vi "AlliGator Generic Graph Actions.vi"(0 "AlliGator Q Elements in":T6[](array[typedef]), 1 "VI in":refnum<vi>, 2 "Script":bool, 5 "data value reference in":refnum<data-value>, 7 "AlliGator Q Event in":T7=enum."GUI:Idle", 9 "Data":variant, 11 "error in (no error)":errorcluster, 12 "AlliGator Ctrl Refnums":T8) -> (3 "Script out":bool, 4 "AlliGator Q Elements out":T6[](array[typedef]), 6 "Data Value Reference out":refnum<data-value>, 10 "[Notebook Message]":T1[](array[typedef]) {"Message Style"."Font Size" min=6.0 step=1.0}, 15 "error out":errorcluster)   [LabVIEW 2021, in "AlliGator Action Engine.lvlib"]
doc: "Processes AlliGator generic graph-related actions."
uses:
  AlliGator Action Engine.lvlib
  Internal Variables/AlliGator Internal Variables v2.ctl
  <vilib>/vision/Image Controls.llb/IMAQ Image.ctl
  Internal Variables/AlliGator Gate Image Set.ctl
  Files/AlliGator FLI Dataset Type.ctl
  Files/AlliGator Data Series Type.ctl
  Dual-Channel Datasets/AlliGator Dataset Channel.ctl
  Settings/AlliGator Gate Arithmetic.ctl
  Source Image/AlliGator Displayed Image.ctl
  Image/Named ROI Description.ctl
  Phasor Graph/AlliGator Decay Metadata v3.ctl
  Decay Analysis/Decay Preprocessing/AlliGator Decay Background Subtraction Info.ctl
  Decay Analysis/Decay Preprocessing/AlliGator Baseline Subtraction Method.ctl
  Graphs/XY Graph/XY Graph Plot Shift Parameters.ctl
  Graphs/XY Graph/XY Graph Plot Shift Method.ctl
  Decay Analysis/Decay Preprocessing/AlliGator Decay Extrapolation Parameters.ctl
  Phasor/Calibration Phasor (m, phi).ctl
  Phasor/Phasor Reference Series.ctl
  Phasor/Phasor Calibration Map v2.ctl
  Phasor/Phasor (g, s).ctl
  Phasor Graph/AlliGator Raw Phasor Plot Data v5.ctl
  Phasor/Phasor Standard Deviation Options.ctl
  Phasor Plot/AlliGator Phasor Multi-Harmonic Data.ctl
  Phasor/Phasor Harmonic Data.ctl
  Decay Fit Parameter Map/AlliGator Decay Fit Options & Parameters v3.ctl
  Fits/IRF(X)PSED/Decay Fit Options v3.ctl
  Fits/Decay Convolution/Decay Model.ctl
  Fits/Residual Type.ctl
  Fits/IRF(X)PSED/Fit Weights Type.ctl
  Fits/Non-linear Fitting Method v2.ctl
  Fits/Fit Calculation Method.ctl
  Fits/Non-linear Fitting Algorithm.ctl
  Decay Analysis/Decay Fit/AlliGator Decay Fit Parameter Constraints 2.ctl
  Fits/IRF(X)PSED/Decay Fit Parameters In List.ctl
  Fits/IRF(X)PSED/MLE Baseline Offset Type.ctl
  Decay Analysis/Decay Preprocessing/AlliGator Decay Preprocessing Parameters.ctl
  Fits/IRF(X)PSED/Decay Fit Parameters & Derived Quantities List v2.ctl
  Fits/IRF(X)PSED/Decay Fit Result Constraint.ctl
  Decay Fit Parameter Map/AlliGator Parameter Maps Data.ctl
  AlliGator Q Event.ctl
  GUI/AlliGator Ctrl Refnums.ctl
  GUI/AlliGator Other Ctrl Refnums.ctl
  GUI/AlliGator State Indicator.ctl
  GUI/AlliGator Main Window Tabs.ctl
  GUI/AlliGator Phasor Plot Ctrl Refnums.ctl
  GUI/AlliGator Phasor Graph Ctrl Refnums.ctl
  Phasor/Phasor Calibration Type.ctl
  GUI/AlliGator Dataset Ctrl Refnums.ctl
  GUI/AlliGator Registered Events Ctrl Refnums.ctl
  GUI/AlliGator Image Histogram Control Refnums.ctl
  Histograms/Linear Histogram Options.ctl
  Histograms/Histogram Bin Option.ctl
  Histograms/Histogram Bin Position.ctl
  Decay Fit Parameter Map/AlliGator Decay Fit Map Control Refnums.ctl
  Parameter Map/AlliGator Parameter Map Control Refnums.ctl
  AlliGator Q Element.ctl
  Notebook/Notebook Message Object.ctl
  Rich Text Box/Text Formatting.ctl
  Rich Text Box/Text Colors.ctl
  Rich Text Box/Text Style.ctl
  Rich Text Box/Text Alignment.ctl
  Graphs/XY Graph/XY Graph Event.ctl
  <vilib>/Utility/miscctls.llb/LVPoint32TypeDef.ctl
  Graphs/XY Graph/XY Graph Mouse Click Event Data.ctl
  Graphs/XY Graph/XY Graph Refnum.ctl
  Rich Text Box/Text Format List.ctl
  Graphs/XY Graph/New Plot Information.ctl
  Graphs/Plot Scales.ctl
  Graphs/LabVIEW Plot Interpolation.ctl
  Graphs/Plot Point Style.ctl
  Graphs/XY Graph/XY Graph Save Plot Data.ctl
  Histograms/Histogram Call Parameters.ctl
  Graphs/XY Graph/XY Graph Add-Ons.lvlib
  Python Plugins API/AlliGator Python Plugins.lvlib
  Graphs/Graphs.lvlib
  Histograms/Histogram Window.lvlib
  Settings/AlliGator Settings.lvlib
  Phasor Graph/AlliGator Phasor Graph.lvlib
  GUI/GUI.lvlib
  Notebook/Notebook.lvlib
  Phasor/Phasor.lvlib
  Image/Image.lvlib
  Decay Analysis/Decay Preprocessing/AlliGator Decay Preprocessing.lvlib
  Files/AlliGator Files.lvlib
  Internal Variables/AlliGator Internal Variables.lvlib
  Phasor Plot/AlliGator Phasor Plot.lvlib
  Source Image/AlliGator Source Image.lvlib
  Fits/Fits.lvlib
  Decay Analysis/Decay Fit/AlliGator Decay Fit.lvlib
  Decay Fit Parameter Map/AlliGator Decay Fit Parameter Map.lvlib
  GUI/AlliGator GUI.lvlib
  Rich Text Box/Rich Text Box.lvlib
  Dual-Channel Datasets/AlliGator Dual-Channel Datasets.lvlib
  Parameter Map/AlliGator Parameter Map.lvlib
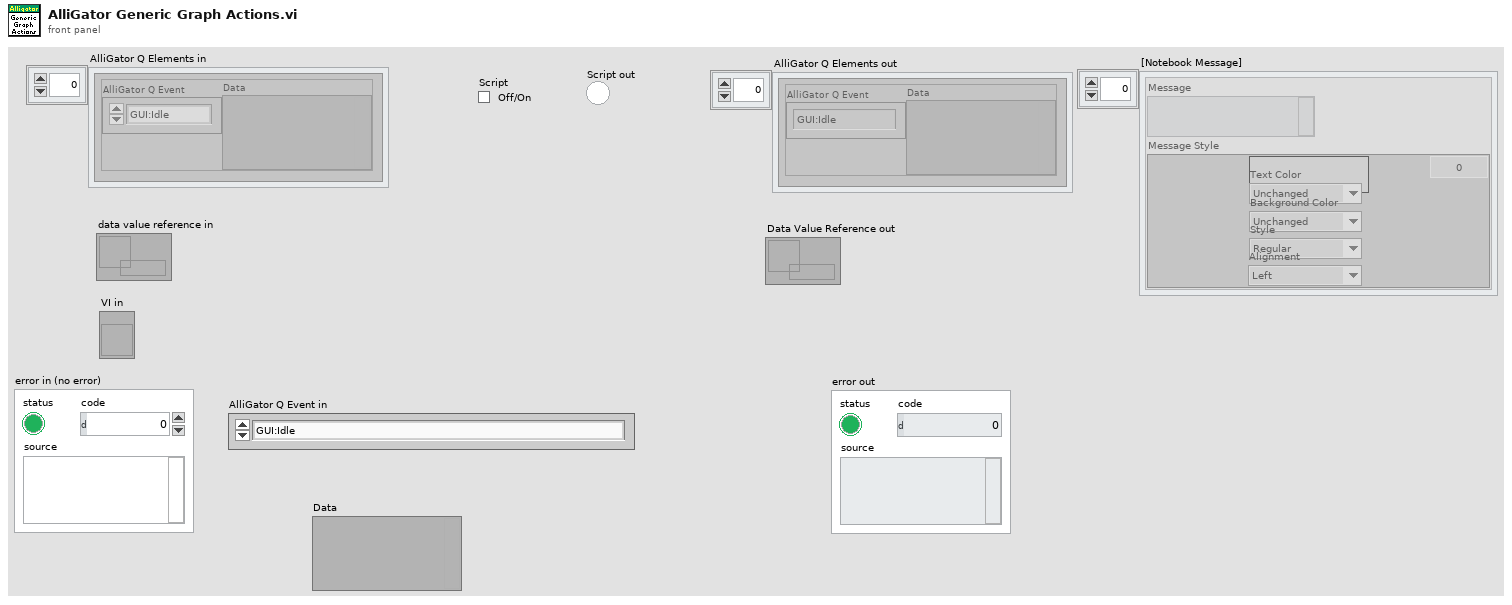
[diagram p1: front panel]
types:
  T1 = typedef "Notebook.lvlib/Notebook Message Object.ctl" = cluster{"Message":string, "Message Style":T2}
  T2 = typedef "Rich Text Box.lvlib/Text Formatting.ctl" = cluster{"Font":string, "Text Color":T3, "Background Color":T3, "Style":T4, "Font Size":dbl, "Alignment":T5}
  T3 = typedef "Rich Text Box.lvlib/Text Colors.ctl" = enum16{"Unchanged", "Black", "Blue", "Cyan", "Maroon", "Gray", "Violet", "Green", "Light Green", "Orange", "Yellow", "Magenta", "Red", "White"}
  T4 = typedef "Rich Text Box.lvlib/Text Style.ctl" = enum16{"Regular", "Bold", "Italic", "Underline", "Strikeout"}
  T5 = typedef "Rich Text Box.lvlib/Text Alignment.ctl" = enum16{"Left", "Right", "Center"}
  T6 = typedef "AlliGator Action Engine.lvlib/AlliGator Q Element.ctl" = cluster{"AlliGator Q Event":T7, "Data":variant}
  T7 = typedef "AlliGator Action Engine.lvlib/AlliGator Q Event.ctl" = enum16{"---- Files ----", "Files:Set Batch Export Files To Save", "Files:Set Dataset Loading & Pre-processing Options", "Files:Check #Frames in Dataset", "Files:Increment Frame Index", "Files:Open Mask Image", "Files:Open White Light Image", "Files:Open Single Dataset", "Files:New Folder of Folders Selected", "Files:Load File (all Types)_Scriptable", "Files:Move Flattened Series to Folders Series", "Files:Select Folder", "Files:Load FLI Dataset", "Files:Load Swiss SPAD 1 Dataset", "Files:Load Swiss SPAD 2 Dataset", "Files:Load .sdt FLI Dataset", "Files:Load .ptu FLI Dataset", "Files:Load .bin FLI Dataset", "Files:Load Single Gate Image Folder", "Files:Load I/m/phi Dataset (deprecated)", "Files:Load Single Image", "Files:Subtract Background File", "Files:Export FLI Dataset", "Files:Load HDF5 FLI Dataset", "Files:Set Destination File Path", "Files:Save Mask Image", "Files:Batch Conversion", "Files:New Folder Selected", "Files:Close FLI Dataset", "Files:Close FLI Dataset Series", "Files:Close White Light Image", "Files:Close Mask Image", "---- FLI Dataset ----", "FLI Dataset:Channel Arithmetic", "FLI Dataset:Export Average Lifetime Map as ASCII", "FLI Dataset:Export User-Defined Quantity Map as ASCII", "FLI Dataset:Python Function FLI Dataset Event", "FLI Dataset:ROI Analysis", "FLI Dataset:Tilted Logistic Square Gated IRF Characteristics Map", "FLI Dataset:Logistic Square Gated IRF Characteristics Map", "FLI Dataset:Square Gated IRF Characteristics Map", "FLI Dataset:Multi-ROI Single-Pixel Phasor Analysis", "FLI Dataset:Multi-ROI Single-Pixel NLSF Analysis", "FLI Dataset:All ROIs IRF Extraction", "FLI Dataset:All ROIs Decay Fit Non-Interactive (Fast + Individual IRF)", "FLI Dataset:All ROIs Phasor Analysis", "FLI Dataset:All ROIs Decay Fit", "FLI Dataset:Fluorescence Decay Statistics", "FLI Dataset:Update Decay Statistics Graph", "FLI Dataset:Get Decay from ROI", "FLI Dataset:All ROIs Average Lifetimes", "FLI Dataset:Save/Load Local IRFs", "FLI Dataset:Clear Local IRFs", "FLI Dataset:Phasor Calibration Maps (# Gates Series) Script", "FLI Dataset:Calibrated Phasor Map Series", "---- FLI Dataset Series ----", "FLI Dataset Series:Sum All Datasets in Series", "FLI Dataset Series:Add Dataset to Accumulated Dataset", "FLI Dataset Series:Display Accumulated Dataset", "FLI Dataset Series:Clear Dataset Series Sum", "FLI Dataset Series:Time-Series Analysis (NLSF)", "FLI Dataset Series:Time-Series Analysis (Phasor)", "---- Image ----", "Image:Update Image Profile Plots", "Image:Image Histogram Cursor Move", "Image:Image Histogram", "Image:Image Contrast", "Image:Set Image Histogram Cursor Move Flag", "Image:Clear Image Overlay", "Image:Use ROI as Search Area", "Image:Set ROI Diameter", "Image:Save Image Data as TIFF", "Image:Save Displayed Image with Overlay", "Image:Save Image Overlay Only", "Image:Save Image as Hot Pixel Mask", "Image:Change Source Image Color Palette", "Image:Copy Image to Clipboard", "Image:Source Image ROI Selection", "Image:Delete All ROIs", "Image:Delete All Unselected ROIs", "Image:Delete ROI", "Image:Merge All ROIs", "Image:Store ROI", "Image:Source Image ROI Storage", "Image:Export ROI Description to Notebook", "Image:Save ROI", "Image:Load ROI", "Image:Paste ROI Definition", "Image:Clear ROI", "Image:Identify ROIs in Mask Image", "Image:Create Complementary ROI", "Image:Create Contour ROI", "Image:Create ROI(s) from Pixels with Peak above Min_Scriptable", "Image:Create ROI(s) from Pixels with Intensity above Min_Scriptable", "Image:Compute ROI Statistics", "Image:Delete ROI(s) based on ROI Characteristics", "Image:Create ROI Grid", "Image:ROI to Individual Pixel ROIs", "Image:Python Function Source Image Event", "Image:Show Phasor Calibration Map ROI Centers", "Image:Convert ROI to Mask Image", "Image:Mouse Move", "Image:Mouse Up", "Image:Set Source Image Mouse Move Flag", "Image:Add Scale Bar Overlay", "Image:Delete Existing ROIs Option", "Image:Overlay ROI Median", "Image:Check Current ROI", "Image:Update True Pixel Value", "---- Decay ----", "Decay:Clear IRF/Reference Plot", "Decay:Add Decay to Graph", "Decay:Smoothen Plot", "Decay:Smoothen Plot Tail", "Decay:Average Selected Plots", "Decay:Extract IRF", "Decay:Optimal IRF Extraction", "Decay:Threshold IRF", "Decay:Fit to Model IRF", "Decay:Fit IRF to Square Gate", "Decay:Fit IRF to Logistic Square Gate", "Decay:Fit IRF to Tilted Logistic Square Gate", "Decay:Create Bounding Cursors Set", "Decay:Export Bounding Cursors Definition to Notebook", "Decay:Denoise Plot", "Decay:Compute Cumulative Function", "Decay:Use as Reference Decay", "Decay:Show Reference Decay/IRF", "Decay:Extrapolate Decay", "Decay:Create Head & Tail Bounding Cursors", "Decay:Store Cursor-defined Head & Tail Fractions", "Decay:Rebin Plot", "Decay:1-Normalize Decay", "Decay:[0-1]-Normalize Plot", "Decay:Straighten Decay", "Decay:Shift Decay", "Decay:Fold Decay", "Decay:Fit Decay", "Decay:Global Fit of Selected Decays", "Decay:Post Global Fit Script", "Decay:Add Global Fit Parameters to Graph", "Decay:Add Decay Parameter(s) to Plot (Graph)", "Decay:Export Decay to Phasor Graph", "Decay:Compute Average Lifetime", "Decay:Plot Convolution", "Decay:Graph Tip Strip Update", "---- Decay Statistics ----", "Decay Statistics:Tip Strip Update", "---- Intensity Time Trace ----", "Intensity Time Trace:Use File Timestamp", "Intensity Time Trace:Load Intensity Corrections File", "Intensity Time Trace:Clear Intensity Corrections File", "Intensity Time Trace:Tip Strip Update", "---- Phasor Plot ----", "Phasor Plot:Build Phasor Plot", "Phasor Plot:Change Phasor Plot Color Palette", "Phasor Plot:Adjust Phasor Plot Display Range", "Phasor Plot:Highlight Image ROI in Phasor Plot", "Phasor Plot:Save Phasor Plot Image with Overlay", "Phasor Plot:Export Complex Phasor Map", "Phasor Plot:Export Phasor Ratio Map", "Phasor Plot:Export Average Lifetime Map", "Phasor Plot:Compute Phase Lifetime Histogram", "Phasor Plot:Compute Phasor Ratio Histogram", "Phasor Plot:Compute Phase Lifetime vs Intensity Scatter Plot", "Phasor Plot:Weber 2-Component Decomposition", "Phasor Plot:Update Phasor Color Map Vertices", "Phasor Plot:Clear Phasor Overlay", "Phasor Plot:Use Segment Extremities as References", "Phasor Plot:Use UC/Segment Intersections as References", "Phasor Plot:Use UC/Principal Axis Intersections as References", "Phasor Plot:Use UC/Linear Fit Intersections as References", "Phasor Plot:Update Phasor Plot Reference", "Phasor Plot:Show Local Phasor Info in Phasor Plot", "Phasor Plot:Update Phasor Plot State", "Phasor Plot:Phasor Plot ROI Storage", "Phasor Plot:Phasor Plot ROI Selection", "Phasor Plot:Python Function Phasor Plot Event", "Phasor Plot:Overlay Phasor ROI, Ratio or Map in Source Image", "Phasor Plot:Compute Decay of Selected Phasors", "Phasor Plot:Phasor at Image Pixel", "Phasor Plot:Mouse Move", "Phasor Plot:Mouse Up", "Phasor Plot:Display Range Mouse Move", "Phasor Plot:Set Mouse Move Flag", "Phasor Plot:Update True Phasor Plot Value", "---- Phasor Graph ----", "Phasor Graph:Get Phasor Value", "Phasor Graph:Create New Phasor Plot Dialog", "Phasor Graph:Update Last Phasor Value", "Phasor Graph:Update Phasor (m, phi)", "Phasor Graph:Remove Single Phasor from Plot", "Phasor Graph:Add Single Phasor to Plot", "Phasor Graph:Remove Phasor Plot", "Phasor Graph:Remove Selected Phasor Plots", "Phasor Graph:Clear Phasor Data", "Phasor Graph:Clear Phasor Graph", "Phasor Graph:Cursor Move", "Phasor Graph:Draw Cursor Connecting Line", "Phasor Graph:Clear Cursor Connecting Line", "Phasor Graph:Find UC Intersection", "Phasor Graph:Use UC/Cursor-Defined Line Intersections", "Phasor Graph:Use Selected Plots Fitted Line/UC Intersections", "Phasor Graph:Use Selected Plots Principal Axis/UC Intersections", "Phasor Graph:Show Single Phasor", "Phasor Graph:Save Single Phasor Plot", "Phasor Graph:Save All Phasor Plots", "Phasor Graph:Load Phasor Plot(s)", "Phasor Graph:Phasor Multiplication", "Phasor Graph:Compute Average Phasor", "Phasor Graph:Compute Multiple Average Phasors (Selected Plots)", "Phasor Graph:Export Single Phasor Plot Phase Lifetimes", "Phasor Graph:Parameter 2 vs Parameter 1 Scatter Plot", "Phasor Graph:Use Cursor n Location", "Phasor Graph:Set Reference n to Current Phase Lifetime Value", "Phasor Graph:Set Reference n to Lifetime Value", "Phasor Graph:Set Cursor n Location", "Phasor Graph:Save Phasor Graph Image", "Phasor Graph:Update SEPL Plot", "Phasor Graph:Export Single Phasor Plot Data", "Phasor Graph:Export Selected Phasor Plots Data", "Phasor Graph:Python Function Phasor Graph Event", "Phasor Graph:Tip Strip Update", "---- Calibration ----", "Calibration:Set Calibration Type", "Calibration:Load/Save Phasor Calibration", "Calibration:Load/Save Phasor Calibration Series", "Calibration:Load/Save Phasor Calibration Map", "Calibration:Use as Calibration", "Calibration:Compute Optimal Calibration from Phasor References", "Calibration:Clear Phasor Calibration", "Calibration:Single Phasor Calibration Information", "Calibration:Use as Calibration Series", "Calibration:Use as Calibration Map", "Calibration:Clear Calibration Series", "Calibration:Phasor Calibration Series Information", "Calibration:Clear Calibration Map", "Calibration:Phasor Calibration Map Information", "Calibration:Apply Phasor Calibration", "Calibration:Update Single Plot Calibration", "Calibration:Update Multiple Plots Calibration", "Calibration:Clear Single Plot Calibration", "Calibration:Clear All Plots Calibrations", "Calibration:Clear Plot(s) Calibration(s)?", "---- Phasor Ratio ----", "Phasor Ratio:Clear Reference n", "Phasor Ratio:Toggle Selected Plot(s)  Lock to Reference 1", "Phasor Ratio:Use as Reference n", "Phasor Ratio:Send Reference n to Notebook", "Phasor Ratio:Toggle Selected Plot(s)  Lock to Reference 2", "Phasor Ratio:Compute Phasor Ratio at Mouse Location", "Phasor Ratio:Compute Phasor Plot's Average Phasor Ratio", "Phasor Ratio:Compute Time-Series Phasor Ratios", "Phasor Ratio:Fit Line to Phasor Ratio Plot", "Phasor Ratio:Save References", "Phasor Ratio:Load References", "Phasor Ratio:Update Phasor Reference 1", "Phasor Ratio:Update Phasor Reference 2", "Phasor Ratio:Move Cursor n to Reference n", "Phasor Ratio:Use as Phasor Reference 1 Lifetime", "Phasor Ratio:Use as Phasor Reference 2 Lifetime", "Phasor Ratio:Export Phasor Ratio Map as ASCII", "Phasor Ratio:Tip Strip Update", "---- Lifetime & Other Parameters Graph ----", "Lifetime:Compute Sliced Mean, SDV and CV Plots", "Lifetime:Plot Decay Shifts", "Lifetime:Plot Histogram", "---- Decay Fit Parameter Map ----", "Decay Fit Parameter Map:Export ROI NLSF Data as ASCII", "Decay Fit Parameter Map:Set Decay Fit Parameter Map Selection", "Decay Fit Parameter Map:Build Decay Fit Parameter Map", "Decay Fit Parameter Map:Change Decay Fit Parameter Map Color Palette", "Decay Fit Parameter Map:Export Decay Fit Parameter Map Data as ASCII", "Decay Fit Parameter Map:Export All Decay Fit Parameter Maps Data as ASCII", "Decay Fit Parameter Map:Selected Parameter Scatterplot", "Decay Fit Parameter Map:Parameter 2 vs Parameter 1 Scatterplot", "Decay Fit Parameter Map:Save Decay Fit Parameter Map Image", "Decay Fit Parameter Map:Save-Load IRFs & Fit Data", "Decay Fit Parameter Map:Update Local Decay Plots", "Decay Fit Parameter Map:Python Function Decay Fit Parameters Map Event", "Decay Fit Parameter Map:Overlay Decay Fit Parameter Map in Source Image", "Decay Fit Parameter Map:Selected Parameter vs Intensity Scatterplot", "Decay Fit Parameter Map:Mouse Up", "Decay Fit Parameter Map:Mouse Move", "Decay Fit Parameter Map:Display Range Mouse Move", "Decay Fit Parameter Map:Change Map Resolution", "Decay Fit Parameter Map:Variance Significance Maps", "Decay Fit Parameter Map:Fit Result Constraints Window", "---- Parameter Map ----", "Parameter Map:Export ROI Parameters Data as ASCII", "Parameter Map:Delete Parameter Map Set", "Parameter Map:Update Parameter List", "Parameter Map:Build Parameter Map", "Parameter Map:Change Parameter Map Color Palette", "Parameter Map:Export Parameter Map Data as ASCII", "Parameter Map:Export All Parameter Maps Data as ASCII", "Parameter Map:Selected Parameter Scatterplot", "Parameter Map:Parameter 2 vs Parameter 1 Scatterplot", "Parameter Map:Selected Parameter vs Intensity Scatterplot", "Parameter Map:Save Parameter Map Image", "Parameter Map:Save-Load IRFs & Parameter Maps (TODO)", "Parameter Map:Set Parameter Map Selection", "Parameter Map:Python Function Parameter Map Event", "Parameter Map:Overlay Parameter Map in Source Image", "Parameter Map:Update Local Decay Plots", "Parameter Map:Mouse Up", "Parameter Map:Mouse Move", "Parameter Map:Display Range Mouse Move", "---- Generic Graph ----", "Generic Graph:Generic XY Graph Event", "Generic Graph:Python Function XY Graph Event", "Generic Graph:New Plot", "Generic Graph:Save Plot", "Generic Graph:XY Plot Histogram", "Generic Graph:Set XY Graph Plot Name", "Generic Graph:Set Last Cursor Style", "Generic Graph:Tip Strip Update", "---- GUI ----", "GUI:Start Script", "GUI:Type of Displayed Image Changed", "GUI:Gate Image Slide Changed", "GUI:Show Busy Icon", "GUI:Show Busy Icon & Abort Button", "GUI:Hide Busy Icon", "GUI:Hide Busy Icon & Abort Button", "GUI:Abort", "GUI:End Script", "GUI:Start Timing", "GUI:End Timing", "GUI:Set State Indicator", "GUI:Send Parameters JSON Strings to Clipboard", "GUI:Set Gate Step", "GUI:Idle", "GUI:Initialization", "GUI:Quit", "GUI:Increment Dataset Index", "GUI:Set Dataset Index to -1", "GUI:Time Series Slider Moved", "GUI:Time Series Slider Changed", "GUI:Toggle Playback or Loop", "GUI:Playback Script", "GUI:Set Phasor Frequency", "GUI:Open Window", "GUI:Start Test Script", "GUI:End Test Script", "GUI:Set Verbose Mode", "GUI:Set Verbose Settings Mode", "DEBUG"}
  T8 = typedef "AlliGator GUI.lvlib/AlliGator Ctrl Refnums.ctl" = cluster{"Other AlliGator Ctrl Refnums":T9, "Phasor Plot Ctrl Refnums":T10, "Phasor Graph Ctrl Refnums":T11, "Dataset Control Refnums":T12, "Registered Events Ctrl Refnums":T13, "Image Histogram Ctrl Refnums":T14, "Decay Fit Map Ctrl Refnums":T15, "Parameter Map Ctrl Refnums":T16}
  T9 = typedef "AlliGator GUI.lvlib/AlliGator Other Ctrl Refnums.ctl" = cluster{"State Indicators":refnum<vi>, " Progress Bar":refnum<vi>, "Decay Graph Active":refnum<vi>, "Decay Statistics Bin":refnum<vi>, "Time Step":refnum<vi>, "Use File Timestamp":refnum<vi>, "Tab Control":refnum<vi>, "CPU":refnum<vi>, "Abort Fit":refnum<vi>, "Dataset File/Folder Path":refnum<vi>, "Abort ROI Creation":refnum<vi>, "Event LED":refnum<vi>, "Dataset File/Folder Path 2":refnum<vi>, "Dataset File/Folder Path 3":refnum<vi>, "Dataset File/Folder Path 4":refnum<vi>, "Dataset File/Folder Path 5":refnum<vi>, "Dataset File/Folder Path 6":refnum<vi>, "Dataset File/Folder Path 7":refnum<vi>, "Dataset File/Folder Path 8":refnum<vi>, "Dataset File/Folder Path 9":refnum<vi>, "Dataset File/Folder Path 10":refnum<vi>, "Dataset File/Folder Path 11":refnum<vi>}
  T10 = typedef "AlliGator GUI.lvlib/AlliGator Phasor Plot Ctrl Refnums.ctl" = cluster{"Phasor Ratio":refnum<vi>, "Modulus Lifetime":refnum<vi>, "Phasor at cursor (m, phi)":refnum<vi>, "Phase Lifetime":refnum<vi>, "Phasor at cursor (g, s)":refnum<vi>, "Phasor Plor Average Lifetime":refnum<vi>, "Phasor Plot Active":refnum<vi>, "Save Phasor Plot":refnum<vi>, "Image Overlay Color":refnum<vi>, "Phasor Plot Color Scale":refnum<vi>, "Reference 1 Button":refnum<vi>, "Reference 2 Button":refnum<vi>, "True Phasor Plot Value":refnum<vi>}
  T11 = typedef "AlliGator GUI.lvlib/AlliGator Phasor Graph Ctrl Refnums.ctl" = cluster{"Phasor Ratio":refnum<vi>, "Modulus Lifetime":refnum<vi>, "Phasor at cursor (m, phi)":refnum<vi>, "Phase Lifetime":refnum<vi>, "Phasor at cursor (g, s)":refnum<vi>, "Phasor Graph Average Lifetime":refnum<vi>, "Phasor Graph Active":refnum<vi>, "Save Phasor Graph":refnum<vi>, "Phasor Frame Slide":refnum<vi>, "Single Step Phasor":refnum<vi>, "Calibration Type":refnum<vi>, "Show Line":refnum<vi>, "Phase Lifetime 1":refnum<vi>, "Phase Lifetime 2":refnum<vi>, "Phasor Graph Frequency":refnum<vi>, "Phasor Reference 1 Control":refnum<vi>, "Phasor Reference 2 Control":refnum<vi>, "Calibration Lifetime":refnum<vi>, "Phase Lifetime SDV":refnum<vi>, "Average Lifetime SDV":refnum<vi>, "Phasor Ratio SDV":refnum<vi>, "Modulus Lifetime SDV":refnum<vi>}
  T12 = typedef "AlliGator GUI.lvlib/AlliGator Dataset Ctrl Refnums.ctl" = cluster{"Current Data":refnum<vi>, "Gate Image Slide":refnum<vi>, "Time Point Slide":refnum<vi>, "Current Time Stamp":refnum<vi>, "Save Image":refnum<vi>, "Displayed Image":refnum<vi>, "Overlay Mode":refnum<vi>, "Phasor Overlay Color":refnum<vi>, "Image Color Scale":refnum<vi>, "Use ROI as Search Area":refnum<vi>, "Source Image ROI Color":refnum<vi>, "True Pixel Value":refnum<vi>}
  T13 = typedef "AlliGator GUI.lvlib/AlliGator Registered Events Ctrl Refnums.ctl" = cluster{"Time Point Slider":refnum<vi>, "Phasor Plot Display Range":refnum<vi>, "Decay Graph":refnum<vi>, "Decay Statistics Graph":refnum<vi>, "Intensity Time Trace":refnum<vi>, "Phasor Graph":refnum<vi>, "Phasor Ratio Graph":refnum<vi>, "Lifetime Graph":refnum<vi>, "Phasor Plot Display":refnum<vi>, "Source Image Display":refnum<vi>, "Decay Fit Parameter Map Display Range":refnum<vi>, "Decay Fit Parameter Map Display":refnum<vi>, "Parameter Map Display Range":refnum<vi>, "Parameter Map Display":refnum<vi>, "Phasor Plot Display Range":refnum<vi>}
  T14 = typedef "AlliGator GUI.lvlib/AlliGator Image Histogram Control Refnums.ctl" = cluster{"Image Histogram":refnum<vi>, "Image Histogram Options":refnum<vi>, "Image Histogram Active":refnum<vi>, "Image Histogram Upper Percentile":refnum<vi>, "Image Histogram Lower Percentile":refnum<vi>, "Auto-Adjust Contrast":refnum<vi>}
  T15 = typedef "AlliGator Decay Fit Parameter Map.lvlib/AlliGator Decay Fit Map Control Refnums.ctl" = cluster{"Decay Fit Parameter Map Color Scale":refnum<vi>, "Decay Fit Parameter":refnum<vi>, "Max Parameter":refnum<vi>, "Min Parameter":refnum<vi>, "Decay Fit Parameter Map Display":refnum<vi>, "Decay Fit Parameter Map Display Range":refnum<vi>, "Decay Parameter Map X":refnum<vi>, "Decay Parameter Map Y":refnum<vi>, "Decay Parameter Map Value":refnum<vi>}
  T16 = typedef "AlliGator Parameter Map.lvlib/AlliGator Parameter Map Control Refnums.ctl" = cluster{"Parameter Map Color Scale":refnum<vi>, "Map Parameter":refnum<vi>, "Max Parameter":refnum<vi>, "Min Parameter":refnum<vi>, "Parameter Map Display":refnum<vi>, "Parameter Map Display Range":refnum<vi>, "Parameter Map Set":refnum<vi>, "Parameter Map X":refnum<vi>, "Parameter Map Y":refnum<vi>, "Parameter Map Value":refnum<vi>}
  T17 = typedef "XY Graph Add-Ons.lvlib/XY Graph Mouse Click Event Data.ctl" = cluster{"Multiplot XY Graph":T18, "Mouse Coordinates":T19}
  T18 = typedef "XY Graph Add-Ons.lvlib/XY Graph Refnum.ctl" = refnum<vi>
  T19 = typedef "LVPoint32TypeDef.ctl" = cluster{"Horizontal":i32, "Vertical":i32}
  T20 = typedef "XY Graph Add-Ons.lvlib/XY Graph Event.ctl" = cluster{"Item Tag":string, "XY Graph Refnum":refnum<vi>, "Coords":T19, "Item Path":string}
  T21 = typedef "Notebook.lvlib/Text Format List.ctl" = enum16{"Message", "Result", "Error", "Setting", "Verbose", "Warning"}
  T22 = typedef "XY Graph Add-Ons.lvlib/New Plot Information.ctl" = cluster{"Multiplot XY Graph":refnum<vi>, "Plot Name":string, "Plot Scales":T23, "Plot Interpolation":T24, "Point Style":T25, "Plot Color":u32, "Plot Metadata":variant}
  T23 = typedef "XY Graph Add-Ons.lvlib/Plot Scales.ctl" = cluster{"X Scale":u32, "Y Scale":u32}
  T24 = typedef "Graphs.lvlib/LabVIEW Plot Interpolation.ctl" = enum16{"Point (.)", "Stepwise Right (--.)", "Line + Point (\\. /)", "Stepwise Left (.--)", "Stepwise Centered (-.-)", "Stepwise Vertical (|.|)", "Line (-)", "Use Previous Plot's Style"}
  T25 = typedef "Graphs.lvlib/Plot Point Style.ctl" = enum16{"not defined", "None", "Empty Circle", "Filled Circle", "Thick Circle", "Dotted Circle", "Empty Square", "Filled Square", "Thick Square", "Dotted Square", "Small Filled Square", "Dot", "Cross", "Tiny Cross", "Large X", "Small x", "Diamond", "Small Empty Square"}
  T26 = typedef "XY Graph Add-Ons.lvlib/XY Graph Save Plot Data.ctl" = cluster{"XY Graph Refnum":refnum<vi>, "Mouse Coords":T19, "File Path":path}
  T27 = typedef "Histogram Window.lvlib/Histogram Call Parameters.ctl" = cluster{"XY Graph Refnum":T18, "Mouse Click Coords":T19, "Plot Index":i32, "Histogram Options":T28}
  T28 = typedef "Histogram Window.lvlib/Linear Histogram Options.ctl" = cluster{"Bin Size":dbl, "Bin Number":i32, "Bin Option":T29, "Min Value":dbl, "Max Value":dbl, "Filter NaN & Infinite Values":bool, "Frequency Plot":bool, "Align Bins":bool, "Bin Location":T30, "Project Outside Values":bool, "Max Histogram Size":i32}
  T29 = typedef "Histogram Window.lvlib/Histogram Bin Option.ctl" = enum32{"Bin Number", "Bin Size"}
  T30 = typedef "Histogram Window.lvlib/Histogram Bin Position.ctl" = enum16{"Left", "Center", "Right"}
  T31 = typedef "XY Graph Add-Ons.lvlib/XY Graph New Plot Name Data.ctl" = cluster{"XY Graph Refnum":T18, "Plot Index":i32, "Plot Name":string, "Allow Duplicate":bool}
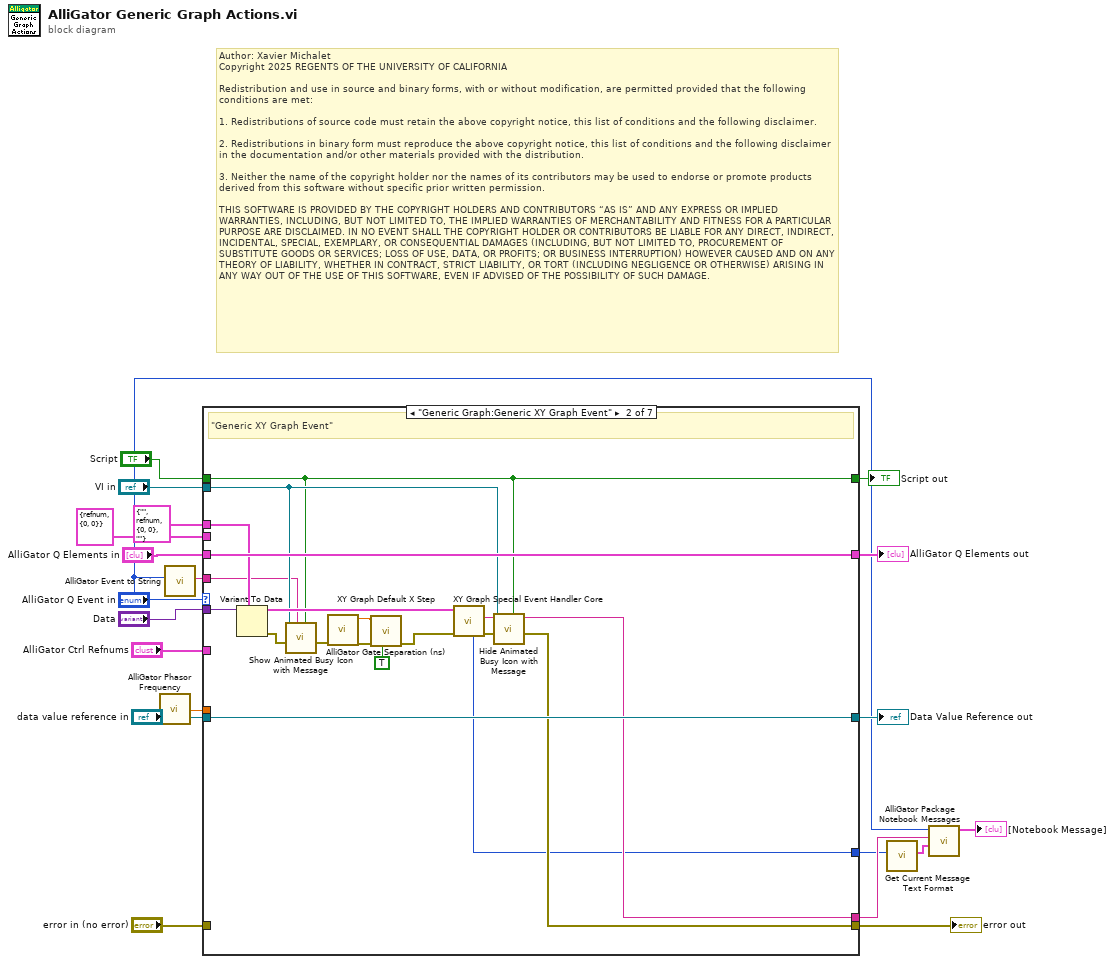
[diagram p0: block diagram]
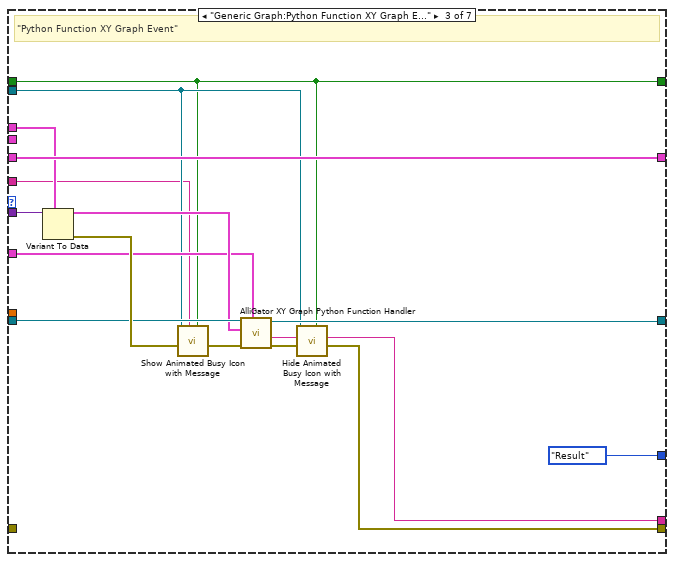
[diagram p3: hidden frame]
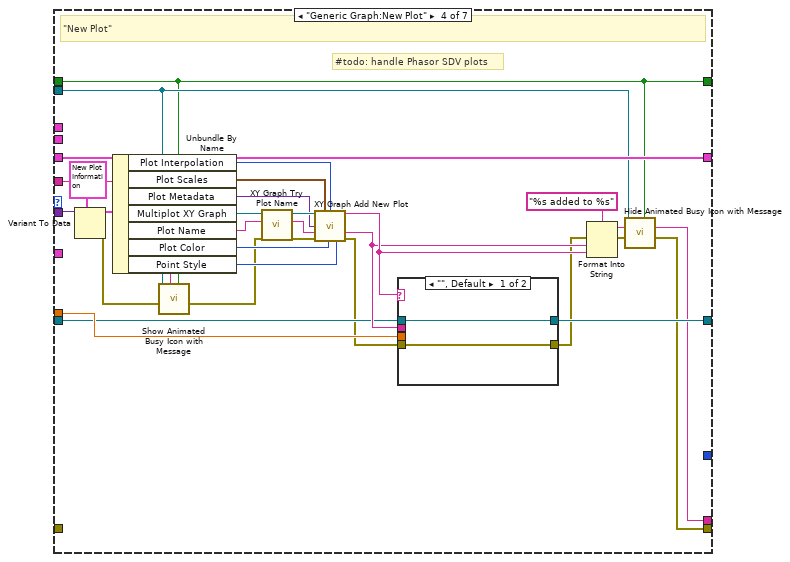
[diagram p4: hidden frame]
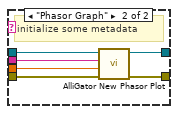
[diagram p5: hidden frame]
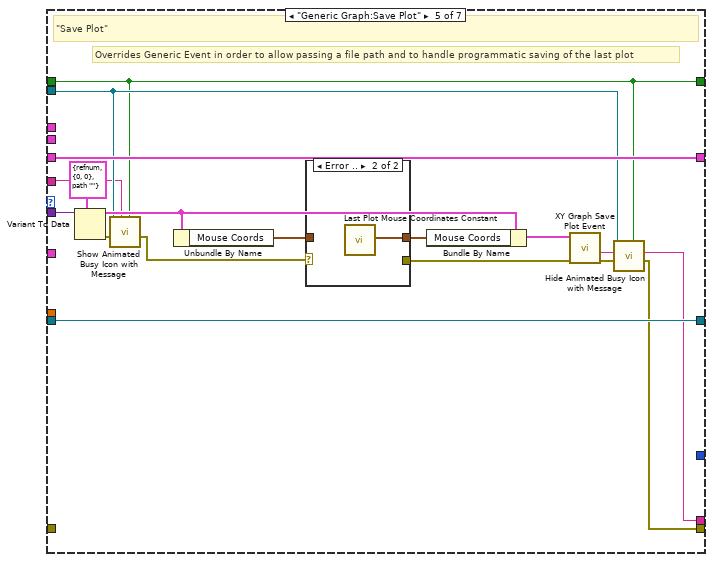
[diagram p6: hidden frame]
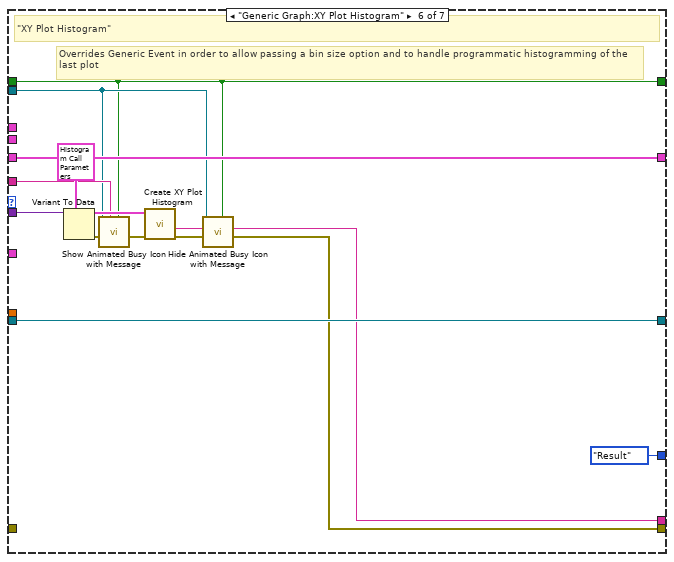
[diagram p8: hidden frame]
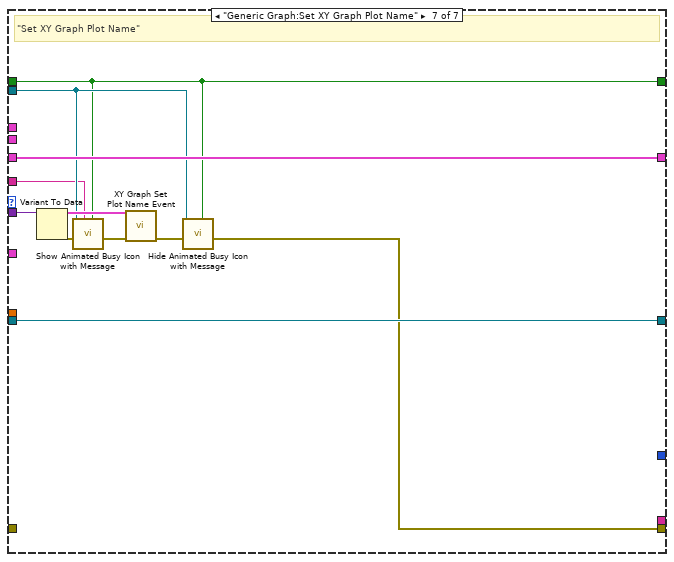
[diagram p9: hidden frame]
diagram:
  # "Author: Xavier Michalet\nCopyright 2025 REGENTS OF THE UNIVERSITY OF CALIFORNIA\n\nRedistribution and use in source and binary forms, with or without modification, are permitted provided that the following conditions are met:\n\n1. Redistributions of source code must retain the above copyright notice, this list of conditions and the following disclaimer.\n\n2. Redistributions in binary form must reproduce the above copyright notice, this list of conditions and the following disclaimer in the documentation and/or other materials provided with the distribution.\n\n3. Neither the name of the copyright holder nor the names of its contributors may be used to endorse or promote products derived from this software without specific prior written permission.\n\nTHIS SOFTWARE IS PROVIDED BY THE COPYRIGHT HOLDERS AND CONTRIBUTORS “AS IS” AND ANY EXPRESS OR IMPLIED WARRANTIES, INCLUDING, BUT NOT LIMITED TO, THE IMPLIED WARRANTIES OF MERCHANTABILITY AND FITNESS FOR A PARTICULAR PURPOSE ARE DISCLAIMED. IN NO EVENT SHALL THE COPYRIGHT HOLDER OR CONTRIBUTORS BE LIABLE FOR ANY DIRECT, INDIRECT, INCIDENTAL, SPECIAL, EXEMPLARY, OR CONSEQUENTIAL DAMAGES (INCLUDING, BUT NOT LIMITED TO, PROCUREMENT OF SUBSTITUTE GOODS OR SERVICES; LOSS OF USE, DATA, OR PROFITS; OR BUSINESS INTERRUPTION) HOWEVER CAUSED AND ON ANY THEORY OF LIABILITY, WHETHER IN CONTRACT, STRICT LIABILITY, OR TORT (INCLUDING NEGLIGENCE OR OTHERWISE) ARISING IN ANY WAY OUT OF THE USE OF THIS SOFTWARE, EVEN IF ADVISED OF THE POSSIBILITY OF SUCH DAMAGE."
  n1 = call "AlliGator Phasor Frequency.vi"() -> ("Phasor Frequency"=w15:dbl[unit])
  n2 = call "AlliGator Event to String.vi"("AlliGator Q Event"="AlliGator Q Event in") -> ("String"=w10:string)  [unwired: 8 in]
  n3 = case shown="\"Generic Graph:Generic XY Graph Event\"" "AlliGator Q Event in" {
    tunnel: "Data" -> [_ w41 w57 w87 w112 w128 w139]
    tunnel: "AlliGator Q Elements in" -> [w24 w42 w58 w86 w111 w129 w140]
    tunnel: [w24 w42 w58 w86 w111 w129 w140] -> w12
    tunnel: "VI in" -> [_ w28 w46 w60 w98 w118 w132]
    tunnel: w15 -> [_ _ _ w74 _ _ _]
    tunnel: "Script" -> [w21 w27 w45 w59 w97 w117 w131]
    tunnel: w10 -> [_ w26 w44 w62 w96 w119 w130]
    tunnel: "error in (no error)" -> [w23 _ _ _ _ _ _]
    tunnel: [w23 w29 w47 w61 w101 w120 w133] -> w9
    tunnel: "AlliGator Ctrl Refnums" -> [_ _ w50 _ _ _ _]
    tunnel: "data value reference in" -> [w22 w38 w54 w73 w106 w123 w135]
    tunnel: [w22 w38 w53 w72 w106 w123 w135] -> w20
    tunnel: [_ w36 w51 w71 w105 w122 _] -> w4
    tunnel: T20 {"Item Tag"="", "XY Graph Refnum"=refnum, "Coords"={"Horizontal"=0, "Vertical"=0}, "Item Path"=""} ("XY Graph Event") -> [_ w35 w49 _ _ _ _]
    tunnel: T17 {"Multiplot XY Graph"=refnum, "Mouse Coordinates"={"Horizontal"=0, "Vertical"=0}} ("Mouse Click Event Data") -> [_ _ _ _ _ _ _]
    tunnel: [w21 w27 w45 w59 w97 w117 w131] -> w6
    tunnel: [_ w25 Text_Format_List."Result" ("Text Format") _ _ Text_Format_List."Result" ("Text Format") _] -> w1
    frame "---- Generic Graph ----", Default {
      # "\"---- Graphs ----\""
    }
    frame "Generic Graph:Generic XY Graph Event" {
      # "\"Generic XY Graph Event\""
      n4 = Variant To Data(type=w35, Variant=w41) -> (data=w39:T20, error out=w37:errorcluster)  [unwired: 1 in]
      n5 = call "Show Animated Busy Icon with Message.vi"("Already active? (F)"=w27, "Message"=w26, "Error In"=w37, "Target VI Refnum"=w28) -> ("Error Out"=w30:errorcluster)  [unwired: 7 in]
      n6 = call "AlliGator Gate Separation (ns).vi"("error in (no error)"=w30) -> ("error out"=w34:errorcluster, "Gate Separation (ns)"=w33:dbl)  [unwired: 9 in]
      n7 = call "XY Graph Default X Step.vi"("Get (F)/Set"=TRUE, "Error In"=w34, "Default X Step"=w33) -> ("Error Out"=w32:errorcluster)  [unwired: 7 in, 1 out]
      n8 = call "XY Graph Special Event Handler Core.vi"("error in (no error)"=w32, "XY Graph Event"=w39) -> ("error out"=w40:errorcluster, "Message"=w36:string, "Message Type"=w25:T21)  [unwired: 4 in, 3 out]
      n9 = call "Hide Animated Busy Icon with Message.vi"("Already active? (F)"=w27, "Error In"=w40, "Target VI reference"=w28) -> ("Error Out"=w29:errorcluster)  [unwired: 8 in]
    }
    frame "Generic Graph:Python Function XY Graph Event" {
      # "\"Python Function XY Graph Event\""
      n10 = Variant To Data(type=w49, Variant=w57) -> (data=w52:T20, error out=w56:errorcluster)  [unwired: 1 in]
      n11 = call "Show Animated Busy Icon with Message.vi"("Already active? (F)"=w45, "Message"=w44, "Error In"=w56, "Target VI Refnum"=w46) -> ("Error Out"=w48:errorcluster)  [unwired: 7 in]
      n12 = call "AlliGator XY Graph Python Function Handler.vi"("AlliGator Ctrl Refnums"=w50, "error in (no error)"=w48, "XY Graph Event"=w52, "data value reference in"=w54) -> ("error out"=w55:errorcluster, "Message"=w51:string, "Data Value Reference out"=w53:refnum<data-value>)  [unwired: 5 in]
      n13 = call "Hide Animated Busy Icon with Message.vi"("Already active? (F)"=w45, "Error In"=w55, "Target VI reference"=w46) -> ("Error Out"=w47:errorcluster)  [unwired: 8 in]
    }
    frame "Generic Graph:New Plot" {
      # "#todo: handle Phasor SDV plots"
      # "\"New Plot\""
      n14 = Variant To Data(type=T22 {"Multiplot XY Graph"=refnum, "Plot Name"="", "Plot Scales"={"X Scale"=0, "Y Scale"=0}, "Plot Interpolation"=enum."Use Previous Plot's Style", "Point Style"=enum."not defined", "Plot Color"=15781887, "Plot Metadata"=variant} ("output cluster"), Variant=w87) -> (data=w85:T22, error out=w83:errorcluster)  [unwired: 1 in]
      n15 = Unbundle By Name(w85) -> ("Plot Interpolation"=w69:T24, "Plot Scales"=w70:T23, "Plot Metadata"=w66:variant, "Multiplot XY Graph"=w81:refnum<vi>, "Plot Name"=w84:string, "Plot Color"=w68:u32, "Point Style"=w67:T25)
      n16 = call "Show Animated Busy Icon with Message.vi"("Already active? (F)"=w59, "Message"=w62, "Error In"=w83, "Target VI Refnum"=w60) -> ("Error Out"=w63:errorcluster)  [unwired: 7 in]
      n17 = call "XY Graph Try Plot Name.vi"("Plot Name in"=w84, "XY Graph Refnum"=w81) -> ("Plot Name out"=w80:string, "XY Graph Refnum"=w79:T18)  [unwired: 6 in, 2 out]
      n18 = call "XY Graph Add New Plot.vi"("Multiplot XY Graph"=w79, "Scales (Default)"=w70, "Plot Interpolation (Previous Plot's Style)"=w69, "Plot Metadata"=w66, "New Plot Name in"=w80, "error in (no error)"=w63, "Plot Color (Default)"=w68, "Point Style (Dot)"=w67) -> ("XY Graph Caption"=w77:string, "New Plot Name out"=w76:string, "error out"=w65:errorcluster)  [unwired: 4 in, 1 out]
      n19 = case shown="\"\", Default" w77 {
        tunnel: w76 -> [_ w95]
        tunnel: w74 -> [_ w94]
        tunnel: w73 -> [w89 w93]
        tunnel: [w89 w92] -> w72
        tunnel: w65 -> [w88 w91]
        tunnel: [w88 w90] -> w64
        frame "", Default {
        }
        frame "Phasor Graph" {
          # "initialize some metadata"
          n20 = call "AlliGator New Phasor Plot.vi"("Error In"=w91, "Phasor Frequency"=w94, "New Plot Name"=w95, "Data Value Reference in"=w93) -> ("Error Out"=w90:errorcluster, "Data Value Reference out"=w92:refnum<data-value>)  [unwired: 6 in]
        }
      }
      n21 = Format Into String(format string="%s added to %s", error in=w64, w76, w77) -> (resulting string=w71:string, error out=w75:errorcluster)  [unwired: 1 in]
      n22 = call "Hide Animated Busy Icon with Message.vi"("Already active? (F)"=w59, "Error In"=w75, "Target VI reference"=w60) -> ("Error Out"=w61:errorcluster)  [unwired: 8 in]
    }
    frame "Generic Graph:Save Plot" {
      # "Overrides Generic Event in order to allow passing a file path and to handle programmatic saving of the last plot"
      # "\"Save Plot\""
      n23 = Variant To Data(type=T26 {"XY Graph Refnum"=refnum, "Mouse Coords"={"Horizontal"=0, "Vertical"=0}, "File Path"=path ""} ("output cluster"), Variant=w112) -> (data=w104:T26, error out=w109:errorcluster)  [unwired: 1 in]
      n24 = call "Show Animated Busy Icon with Message.vi"("Already active? (F)"=w97, "Message"=w96, "Error In"=w109, "Target VI Refnum"=w98) -> ("Error Out"=w100:errorcluster)  [unwired: 7 in]
      n25 = Unbundle By Name(w104) -> ("Mouse Coords"=w108:T19)
      n26 = case shown="Error .." w100 {
        selector: w100 -> [w113 _]
        tunnel: w108 -> [w114 _]
        tunnel: [w114 w115] -> w103
        tunnel: [w113 _] -> w99
        frame No Error {
        }
        frame Error {
          n27 = call "Last Plot Mouse Coordinates Constant.vi"() -> ("Selected Plots Mouse Coordinates Equivalent"=w115:T19)
        }
      }
      n28 = Bundle By Name(cluster=w104, "Mouse Coords"=w103) -> (w102:T26)
      n29 = call "XY Graph Save Plot Event.vi"("Error In"=w99, "AliGator Save Plot Data"=w102) -> ("Error Out"=w110:errorcluster, "Message"=w105:string)  [unwired: 4 in, 4 out]
      n30 = call "Hide Animated Busy Icon with Message.vi"("Already active? (F)"=w97, "Error In"=w110, "Target VI reference"=w98) -> ("Error Out"=w101:errorcluster)  [unwired: 8 in]
    }
    frame "Generic Graph:XY Plot Histogram" {
      # "Overrides Generic Event in order to allow passing a bin size option and to handle programmatic histogramming of the last plot"
      # "\"XY Plot Histogram\""
      n31 = Variant To Data(type=T27 {"XY Graph Refnum"=refnum, "Mouse Click Coords"={"Horizontal"=0, "Vertical"=0}, "Plot Index"=-1, "Histogram Options"={"Bin Size"=0.0, "Bin Number"=0, "Bin Option"=enum."Bin Number", "Min Value"=-inf, "Max Value"=inf, "Filter NaN & Infinite Values"=TRUE, "Frequency Plot"=FALSE, "Align Bins"=FALSE, "Bin Location"=enum."Left", "Project Outside Values"=FALSE, "Max Histogram Size"=100000}} ("Plot Histogram Call Parameters"), Variant=w128) -> (data=w127:T27, error out=w126:errorcluster)  [unwired: 1 in]
      n32 = call "Show Animated Busy Icon with Message.vi"("Already active? (F)"=w117, "Message"=w119, "Error In"=w126, "Target VI Refnum"=w118) -> ("Error Out"=w121:errorcluster)  [unwired: 7 in]
      n33 = call "Create XY Plot Histogram.vi"("error in (no error)"=w121, "Plot Histogram Call Parameters"=w127) -> ("error out"=w125:errorcluster, "Message"=w122:string)  [unwired: 7 in, 1 out]
      n34 = call "Hide Animated Busy Icon with Message.vi"("Already active? (F)"=w117, "Error In"=w125, "Target VI reference"=w118) -> ("Error Out"=w120:errorcluster)  [unwired: 8 in]
    }
    frame "Generic Graph:Set XY Graph Plot Name" {
      # "\"Set XY Graph Plot Name\""
      n35 = Variant To Data(Variant=w139) -> (data=w138:T31, error out=w137:errorcluster)  [unwired: 2 in]
      n36 = call "Show Animated Busy Icon with Message.vi"("Already active? (F)"=w131, "Message"=w130, "Error In"=w137, "Target VI Refnum"=w132) -> ("Error Out"=w134:errorcluster)  [unwired: 7 in]
      n37 = call "XY Graph Set Plot Name Event.vi"("Error In"=w134, "Plot Name Data"=w138) -> ("Error Out"=w136:errorcluster)  [unwired: 9 in]
      n38 = call "Hide Animated Busy Icon with Message.vi"("Already active? (F)"=w131, "Error In"=w136, "Target VI reference"=w132) -> ("Error Out"=w133:errorcluster)  [unwired: 8 in]
    }
  }
  "Data Value Reference out" <- w20
  "error out" <- w9
  "AlliGator Q Elements out" <- w12
  "Script out" <- w6
  n39 = call "Get Current Message Text Format.vi"("Text Format"=w1) -> ("Message Formatting"=w3:T2)  [unwired: 8 in, 1 out]
  n40 = call "AlliGator Package Notebook Messages.vi"("Message Formatting"=w3, "Message"=w4, "AlliGator Q Event in"="AlliGator Q Event in") -> ("[Notebook Message]"=→"[Notebook Message]":T1[])  [unwired: 8 in]
